vi "ExampleQueryServer.vi"() -> ()   [LabVIEW 2019]
uses:
  VIs/labview-grpc-query-server.lvlib
  gRPC interface/gprc-lvsupport.lvlib
panel:
  in  "Server Key File (.key)":path
  in  "Server Certificate File (.crt)":path
  in  "stop":bool
  in  "Server Address":string="0.0.0.0:50051"
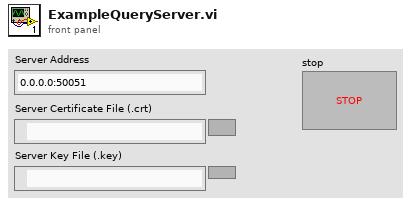
[diagram p1: front panel]
types:
  T1 = typedef "gprc-lvsupport.lvlib/grpcId.ctl" = u64
  T2 = cluster{"QueryServer_Invoke":refnum<user-event>, "QueryServer_Query":refnum<user-event>, "QueryServer_Register":refnum<user-event>, "serverId":T1}
  T3 = typedef "gprc-support.lvlib/grpcId.ctl" = u64
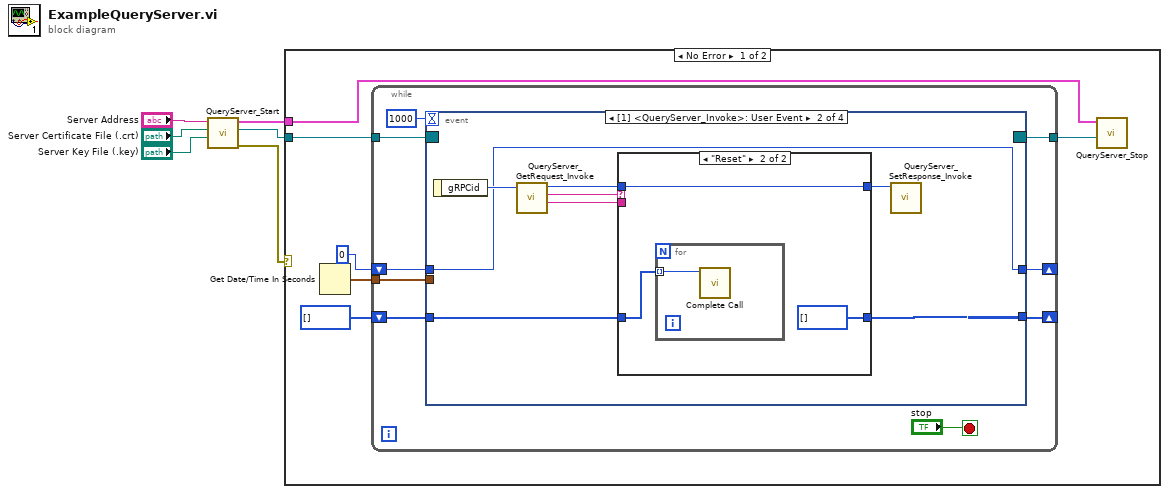
[diagram p0: block diagram]
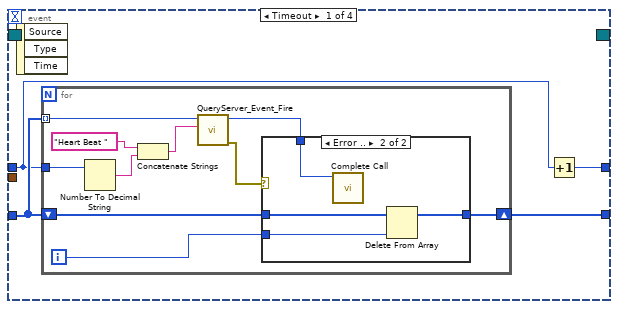
[diagram p2: hidden frame]
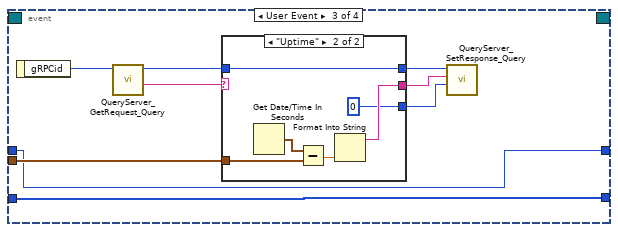
[diagram p5: hidden frame]
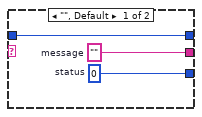
[diagram p6: hidden frame]
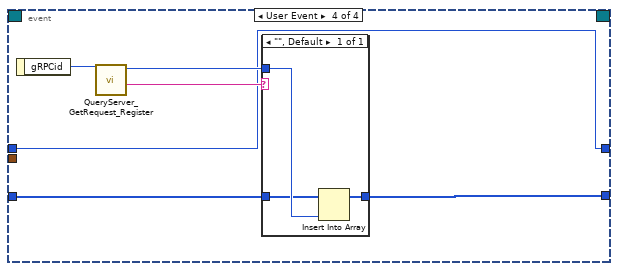
[diagram p7: hidden frame]
diagram:
  n1 = call "QueryServer_Start.vi"("Server Key File (.key)"="Server Key File (.key)", "Server Certificate File (.crt)"="Server Certificate File (.crt)", "Server Address"="Server Address") -> ("error out"=w2:errorcluster, "Event Registration Refnum"=w1:refnum<event-registration>, "Server Info"=w5:T2)  [unwired: 5 in]
  n2 = case shown="No Error" w2 {
    tunnel: w5 -> [w10 _]
    tunnel: w1 -> [w8 _]
    frame No Error {
      n3 = Get Date/Time In Seconds() -> (seconds since 1Jan1904=w12:timestamp)
      n4 = while {
        tunnel: [w20] -> w9
        tunnel: w12 -> [w19]
        shift-right: [w17] -> _
        shift-left: u64[] [] -> [w16]
        tunnel: w8 -> [w15]
        shift-right: [w13] -> _
        shift-left: 0 -> [w14]
        stop <- "stop" stop-if-true
        n5 = event shown="[1] <QueryServer_Invoke>: User Event" {
          selector: w15 -> [_ _ _ _]
          dyn-events: [_ _ _ _] -> w20
          timeout: 1000 -> [_ _ _ _]
          tunnel: w19 -> [_ _ w58 _]
          tunnel: [w24 w42 w57 w76] -> w17
          tunnel: w16 -> [w25 w43 w57 w75]
          tunnel: w14 -> [w23 w41 w55 w73]
          tunnel: [w22 w41 w55 w73] -> w13
          event Timeout {
            n6 = event-data() -> ()  [unwired: 1 in, 3 out]
            n7 = for {
              tunnel: w25 -> [w35] mode=indexing
              shift-right: [w32] -> w24
              shift-left: w25 -> [w31]
              tunnel: w23 -> [w26]
              i -> [w33]
              n8 = Number To Decimal String(number=w26) -> (decimal integer string=w29:string)  [unwired: 1 in]
              n9 = Concatenate Strings("Heart Beat " ("eventdata"), w29) -> (w27:string)
              n10 = call "QueryServer_Event_Fire.vi"("eventdata"=w27, "gRPCid"=w35) -> ("error out"=w34:errorcluster, "gRPCid out"=w30:T1)  [unwired: 8 in]
              n11 = case shown="Error .." w34 {
                tunnel: w31 -> [w36 w40]
                tunnel: w33 -> [_ w39]
                tunnel: [w36 w38] -> w32
                tunnel: w30 -> [_ w37]
                frame No Error {
                }
                frame Error {
                  n12 = call "Complete Call.vi"("gRPCid"=w37) -> ()  [unwired: 9 in, 1 out]
                  n13 = Delete From Array(array=w40, index=w39) -> (array with subset deleted=w38:u64[])  [unwired: 1 in, 1 out]
                }
              }
            }
            n14 = Increment(x=w23) -> (x+1=w22:i32)
          }
          event User Event {
            n15 = event-data() -> ("gRPCid"=w48:T3)  [unwired: 1 in]
            n16 = call "QueryServer_GetRequest_Invoke.vi"("gRPCid"=w48) -> ("parameter"=w44:string, "command"=w47:string, "gRPCid out"=w46:T1)  [unwired: 5 in, 1 out]
            n17 = case shown="\"Reset\"" w47 {
              tunnel: w46 -> [w50 w51]
              tunnel: [w50 w51] -> w45
              tunnel: w44 -> [_ _]
              tunnel: w43 -> [w49 w53]
              tunnel: [w49 u64[] []] -> w42
              frame "", Default {
              }
              frame "Reset" {
                n18 = for {
                  tunnel: w53 -> [w54] mode=indexing
                  n19 = call "Complete Call.vi"("gRPCid"=w54) -> ()  [unwired: 9 in, 1 out]
                }
              }
            }
            n20 = call "QueryServer_SetResponse_Invoke.vi"("gRPCid"=w45) -> ()  [unwired: 9 in, 1 out]
          }
          event User Event {
            n21 = event-data() -> ("gRPCid"=w63:T3)  [unwired: 1 in]
            n22 = call "QueryServer_GetRequest_Query.vi"("gRPCid"=w63) -> ("gRPCid out"=w62:T1, "query"=w56:string)  [unwired: 7 in, 1 out]
            n23 = case shown="\"Uptime\"" w56 {
              tunnel: w62 -> [w66 w68]
              tunnel: [w66 w68] -> w61
              tunnel: [w65 w69] -> w60
              tunnel: [w64 0 ("status")] -> w59
              tunnel: w58 -> [_ w71]
              frame "", Default {
                w64 = 0  # status
                w65 = ""  # message
              }
              frame "Uptime" {
                n24 = Get Date/Time In Seconds() -> (seconds since 1Jan1904=w72:timestamp)
                n25 = Subtract(x=w72, y=w71) -> (x-y=w70:dbl)
                n26 = Format Into String(w70) -> (resulting string=w69:string)  [unwired: 3 in, 1 out]
              }
            }
            n27 = call "QueryServer_SetResponse_Query.vi"("gRPCid"=w61, "message"=w60, "status"=w59) -> ()  [unwired: 7 in, 1 out]
          }
          event User Event {
            n28 = event-data() -> ("gRPCid"=w78:T3)  [unwired: 1 in]
            n29 = call "QueryServer_GetRequest_Register.vi"("gRPCid"=w78) -> ("gRPCid out"=w77:T1, "eventname"=w74:string)  [unwired: 7 in, 1 out]
            n30 = case shown="\"\", Default" w74 {
              tunnel: w77 -> [w81]
              tunnel: [w80] -> w76
              tunnel: w75 -> [w79]
              frame "", Default {
                n31 = Insert Into Array(array=w79, new element=w81) -> (w80:u64[])  [unwired: 1 in]
              }
            }
          }
        }
      }
      n32 = call "QueryServer_Stop.vi"("Server Info"=w10, "Event Registration Refnum"=w9) -> ()  [unwired: 8 in, 1 out]
    }
    frame Error {
    }
  }
